vi "find_consecutive_close_data_with_a_reference.vi"(7 "Python module path":path, 8 "error in (no error)":errorcluster, 9 "Tol %":dbl format="%.2f", 10 "Ref [W]":dbl format="%.2f", 11 "data":dbl[](array[numeric])) -> (0 "error out":errorcluster, 1 "# elements found":i32, 2 "data qty":i32, 3 "Measures":dbl[][](array[numeric]), 4 "close values":dbl[](array[numeric]), 5 "average":dbl)   [LabVIEW 2024]
panel:
  out "Plot":dbl[][](graph)
  # "Measurements found in range"
  # "Powered by \nPython 3.9.13\n32-bits"
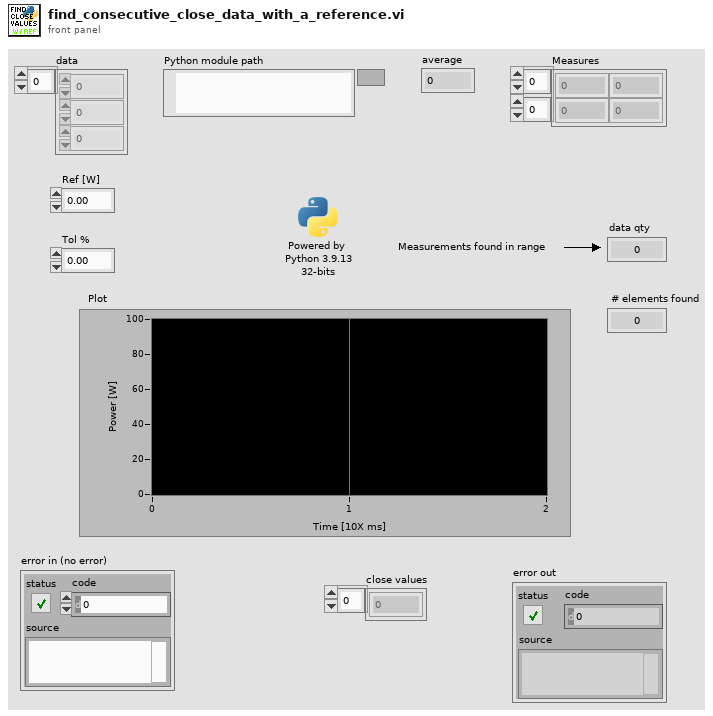
[diagram p1: front panel]
types:
  T1 = cluster{"close values w zero":dbl[], "# elements found":i32, "close values":dbl[], "average":dbl}
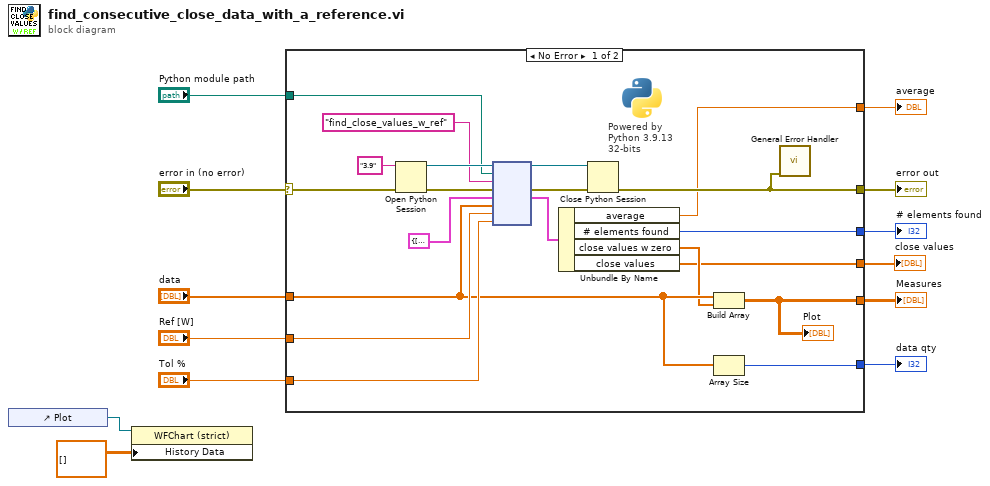
[diagram p0: block diagram]
diagram:
  n1 = control-ref of="Plot"() -> (w8:refnum<vi>)
  n2 = property class="WFChart (strict)"(reference=w8, "History Data"=dbl[][] []) -> ()  [unwired: 1 in, 2 out]
  n3 = case shown="No Error" "error in (no error)" {
    selector: "error in (no error)" -> [w23 w34]
    tunnel: "Ref [W]" -> [w28 _]
    tunnel: "Tol %" -> [w27 _]
    tunnel: [w26 _] -> w9
    tunnel: [w18 _] -> w11
    tunnel: [w15 w34] -> w10
    tunnel: "data" -> [w20 _]
    tunnel: [w21 _] -> w4
    tunnel: [w14 _] -> w3
    tunnel: [w17 _] -> w2
    tunnel: "Python module path" -> [w16 _]
    frame No Error {
      # "Powered by \nPython 3.9.13\n32-bits"
      n4 = Open Python Session(python version="3.9" ("Python version"), 3:w23) -> (session out=w33:refnum<k35>, error out=w22:errorcluster)  [unwired: 1 in]
      n5 = node(w33, w16, "find_close_values_w_ref" ("function name"), w22, T1 {"close values w zero"=[], "# elements found"=0, "close values"=[], "average"=0.0}, w20, w28, w27) -> (w30:refnum<k35>, w31:errorcluster, w24:T1)  [unwired: 3 in, 2 out]
      n6 = Unbundle By Name(w24) -> ("average"=w14:dbl, "# elements found"=w18:i32, "close values w zero"=w19:dbl[], "close values"=w17:dbl[])
      n7 = Close Python Session(session in=w30, error in=w31) -> (11:w15:errorcluster)
      n8 = Build Array(w20, w19) -> (w26:dbl[][])
      "Plot" <- w26
      n9 = Array Size(array=w20) -> (size(s)=w21:i32)
      n10 = call <vilib>:"General Error Handler.vi"("error in (no error)"=w15) -> ()  [unwired: 10 in, 5 out]
    }
    frame Error {
    }
  }
  "# elements found" <- w11
  "error out" <- w10
  "Measures" <- w9
  "data qty" <- w4
  "average" <- w3
  "close values" <- w2
